vi "ReadDefaultSchedules.vi"(10 "File Name":string) -> (0 "Times Called":dbl, 1 "Scheduler":T1(array[cluster]), 2 "File Exists":bool)   [LabVIEW 2018]
panel:
  out "Numeric":dbl
  out "File Path":path
  in  "Path":path
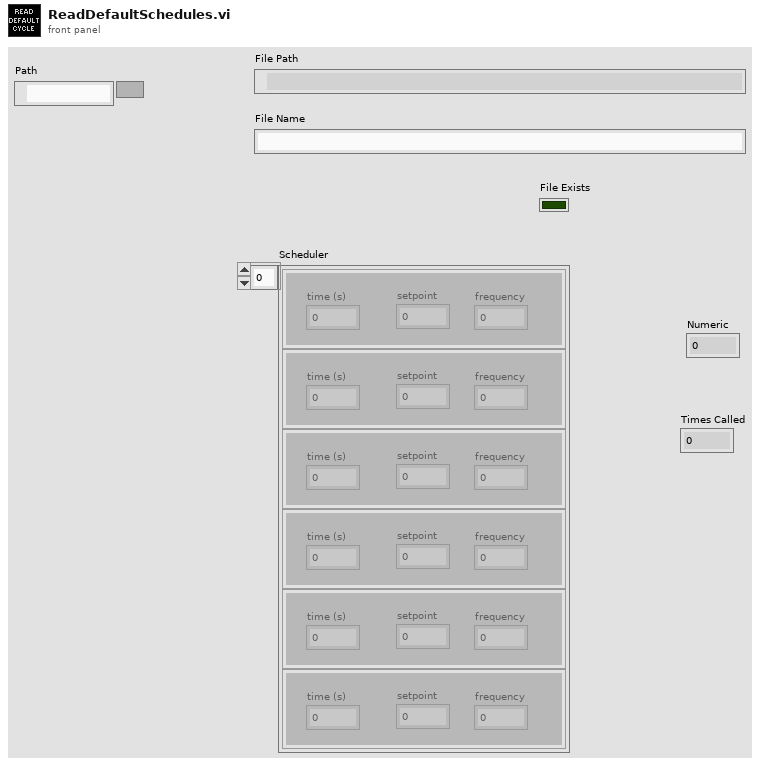
[diagram p1: front panel]
types:
  T1 = cluster{"time (s)":dbl, "setpoint ":dbl, "frequency":dbl}[]
  T2 = cluster{"[0]":dbl, "[1]":dbl, "[2]":dbl, "[3]":dbl, "[4]":dbl, "[5]":dbl, "[6]":dbl, "[7]":dbl, "[8]":dbl}
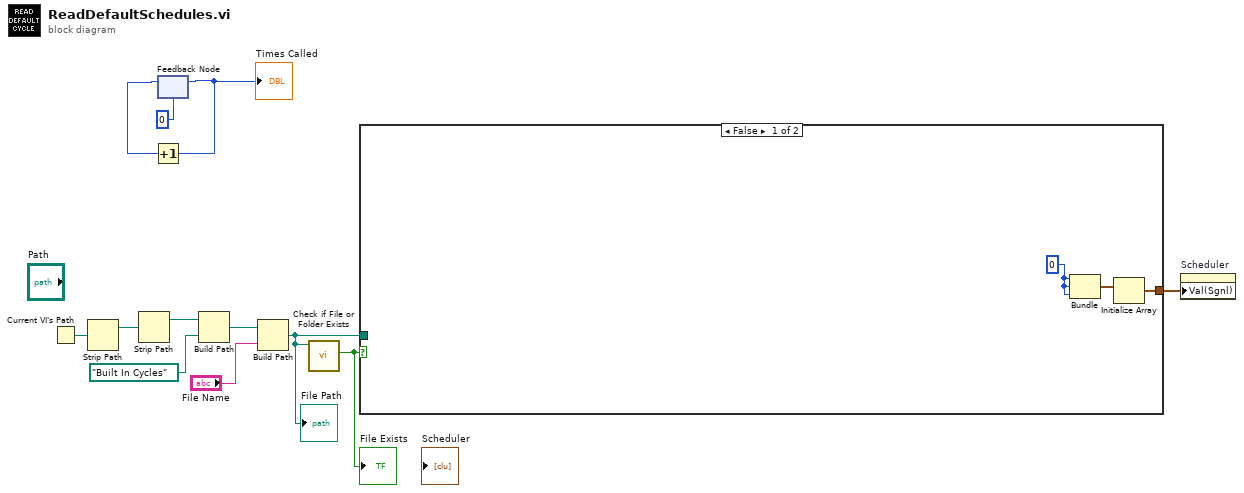
[diagram p0: block diagram]
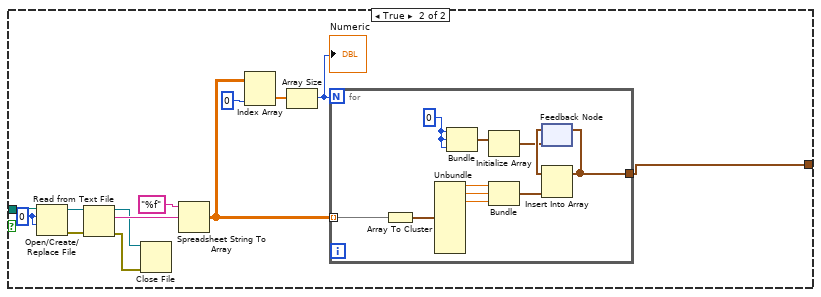
[diagram p2: hidden frame]
diagram:
  n1 = Current VI's Path() -> (path=w8:path)
  n2 = Strip Path(path=w8) -> (stripped path=w9:path)  [unwired: 1 out]
  n3 = Strip Path(path=w9) -> (stripped path=w11:path)  [unwired: 1 out]
  n4 = feedback #1(0) -> (w2:i32)
  n5 = Increment(x=w2) -> (x+1=w1:i32)
  "Times Called" <- w1
  n6 = feedback-in #1(w1) -> ()
  n7 = Build Path(base path=w11, name or relative path=path "Built In Cycles") -> (appended path=w10:path)
  n8 = Build Path(base path=w10, name or relative path="File Name") -> (appended path=w5:path)
  "File Path" <- w5
  n9 = call <vilib>:"Check if File or Folder Exists.vi"("path"=w5) -> ("file or folder exists?"=w6:bool)  [unwired: 8 in, 2 out]
  "File Exists" <- w6
  n10 = case shown="False" w6 {
    tunnel: w5 -> [_ w17]
    tunnel: [w13 w22] -> w4
    frame False {
      w15 = 0
      n11 = Bundle(w15, w15, w15) -> (w14:cluster{i32, i32, i32})  [unwired: 1 in]
      n12 = Initialize Array(w14) -> (w13:cluster{i32, i32, i32}[])  [unwired: 1 in]
    }
    frame True {
      w16 = 0
      n13 = Open/Create/Replace File(file path (use dialog)=w17, operation (0:open)=w16, access (0:read/write)=w16) -> (refnum out=w18:refnum<file>, error out=w20:errorcluster)  [unwired: 3 in, 1 out]
      n14 = Read from Text File(file (use dialog)=w18, error in=w20) -> (refnum out=w21:refnum<file>, text=w28:string, error out=w19:errorcluster)  [unwired: 2 in, 1 out]
      n15 = Close File(refnum=w21, error in=w19) -> ()  [unwired: 2 out]
      n16 = Spreadsheet String To Array(format string="%f", spreadsheet string=w28) -> (array=w26:dbl[][])  [unwired: 2 in]
      n17 = Index Array(array=w26, index (col)=0) -> (element=w25:dbl[])  [unwired: 1 in]
      n18 = Array Size(array=w25) -> (size(s)=w23:i32)
      "Numeric" <- w23
      n19 = for {
        N: w23 -> [_]
        tunnel: w26 -> [w39] mode=indexing
        tunnel: [w32] -> w22
        w30 = 0
        n20 = Array To Cluster(array=w39) -> (cluster=w38:T2)
        n21 = Unbundle(w38) -> ("[0]"=w37:dbl, "[1]"=w36:dbl, "[2]"=w35:dbl)  [unwired: 6 out]
        n22 = Bundle(w30, w30, w30) -> (w31:cluster{i32, i32, i32})  [unwired: 1 in]
        n23 = Initialize Array(w31) -> (w29:cluster{i32, i32, i32}[])  [unwired: 1 in]
        n24 = Bundle("[0]"=w37, "[1]"=w36, "[2]"=w35) -> (w34:cluster{"[0]":dbl, "[1]":dbl, "[2]":dbl})  [unwired: 1 in]
        n25 = feedback #2(w29) -> (w33:cluster{i32, i32, i32}[])
        n26 = Insert Into Array(array=w33, new element=w34) -> (w32:cluster{i32, i32, i32}[])  [unwired: 1 in]
        n27 = feedback-in #2(w32) -> ()
      }
    }
  }
  n28 = property on="Scheduler" class="Arr (strict)"("Val(Sgnl)"=w4) -> ()  [unwired: 2 in, 2 out]
